vi "GenerateTimeAndDateCSV.vi"(11 "Test string input":string) -> (3 "path for csv file":path)   [LabVIEW 2020, in "WritingDataFile.lvlib"]
uses:
  WritingDataFile.lvlib
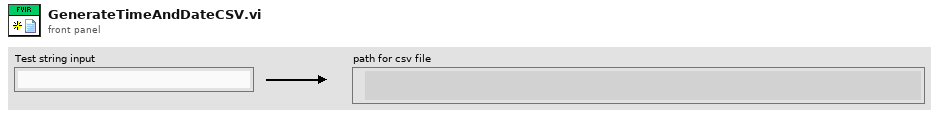
[diagram p1: front panel]
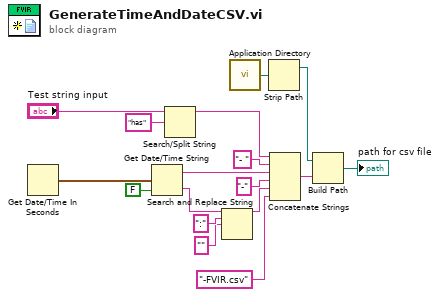
[diagram p0: block diagram]
diagram:
  n1 = Get Date/Time In Seconds() -> (seconds since 1Jan1904=w10:timestamp)
  n2 = Get Date/Time String(seconds (now)=w10, want seconds? (F)=FALSE) -> (date string=w3:string, time string=w12:string)  [unwired: 1 in]
  n3 = Search/Split String(string="Test string input", search string/char (-)="has") -> (substring before match=w13:string)  [unwired: 1 in, 2 out]
  n4 = Search and Replace String(input string=w12, search string=":", replace string="" ("replace string (\"\")")) -> (result string=w16:string)  [unwired: 5 in, 3 out]
  n5 = call <vilib>:"Application Directory.vi"() -> ("Application Directory"=w8:path)
  n6 = Strip Path(path=w8) -> (stripped path=w9:path)  [unwired: 1 out]
  n7 = Concatenate Strings(w13, "- ", w3, "-" ("string"), w16, "-FVIR.csv" ("string")) -> (w15:string)
  n8 = Build Path(base path=w9, name or relative path=w15) -> (appended path=→"path for csv file":path)
